vi "Write Transmission Data Unit.vi"(8 "error in":errorcluster, 10 "transmission data unit":refnum<class "Transmission Data Unit.lvclass">, 11 "Modbus instance in":refnum<class "Modbus API.lvclass">) -> (0 "error out":errorcluster, 3 "Modbus instance out":refnum<class "Modbus API.lvclass">)   [LabVIEW 2013, in "Modbus Library - Advance.lvlib" / "Modbus API.lvclass"]
doc: "This VI is an accessor for the transmission data unit stored in the modbus instance. This accessor can be used as a property node. The transmission data unit is used by the device to determine how to pack and unpack data coming from the physical bus."
uses:
  Modbus API.lvclass
  Transmission Data Unit/Transmission Data Unit.lvclass
  Modbus API.lvclass/Modbus API.ctl
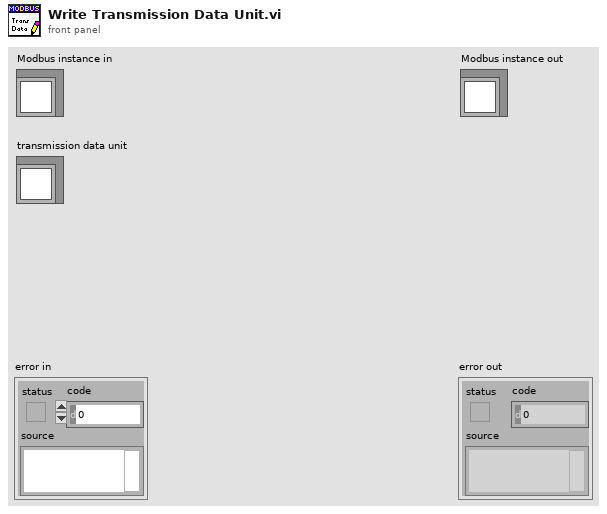
[diagram p1: front panel]
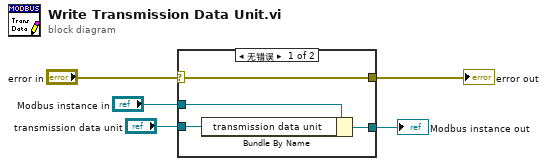
[diagram p0: block diagram]
diagram:
  n1 = case shown="无错误" "error in" {
    selector: "error in" -> [w9 w10]
    tunnel: [w9 w10] -> w4
    tunnel: [w7 w11] -> w2
    tunnel: "Modbus instance in" -> [w8 w11]
    tunnel: "transmission data unit" -> [w6 _]
    frame No Error {
      n2 = Bundle By Name(cluster=w8, "transmission data unit"=w6) -> (w7:refnum<class "Modbus API.lvclass">)
    }
    frame Error {
    }
  }
  "error out" <- w4
  "Modbus instance out" <- w2
